vi "Corners to Rectangle.vi"(10 "Corners 2":cluster{"X":sgl, "Y":sgl}[](array[cluster])=[{"X"=418.12665, "Y"=424.52673}, {"X"=459.83737, "Y"=432.6989}, {"X"=455.7626, "Y"=481.78384}, {"X"=413.9875, "Y"=474.98163}, {"X"=418.12665, "Y"=424.52673}]) -> (2 "output cluster":T1, 4 "Aspect Ratio":sgl, 5 "Center":cluster{"X":dbl, "Y":dbl} {"Y" format="%0.2f"; "X" format="%0.2f"})   [LabVIEW 2023]
uses:
  Target Fields.ctl
  <vilib>/Analysis/baseanly.llb/Mean (DBL).vi
  <vilib>/Analysis/NI_AALBase.lvlib
panel:
  out "Tilted Left/Right":bool
  out "Tilted Up/down":bool
  out "Vert Size":sgl
  out "Horz Size":sgl
  out "Rectangle":T2
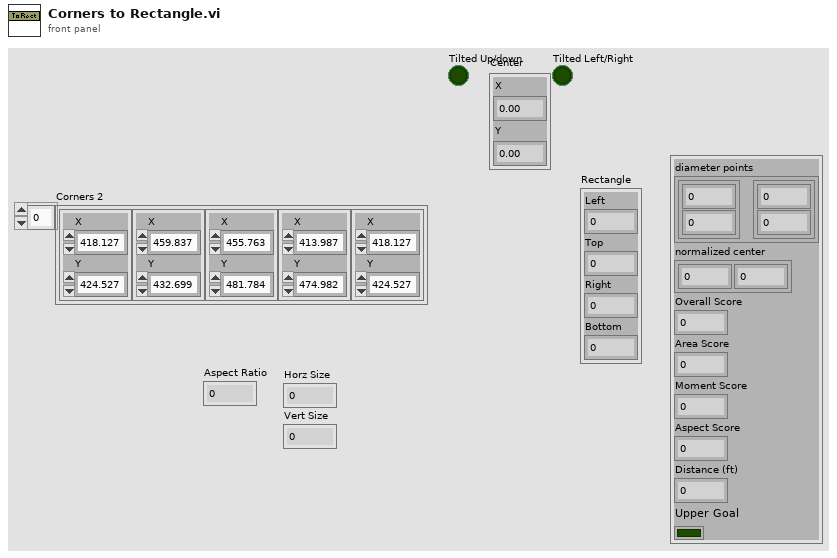
[diagram p1: front panel]
types:
  T1 = typedef "Target Fields.ctl" = cluster{"diameter points":cluster{"first point":cluster{"x":dbl, "y":dbl}, "projected point":cluster{"x":dbl, "y":dbl}}, "normalized center":cluster{"x":dbl, "y":dbl}, "Overall Score":dbl, "Area Score":dbl, "Moment Score":dbl, "Aspect Score":dbl, "Distance (ft)":dbl, "Upper Goal":bool}
  T2 = cluster{"Left":i32, "Top":i32, "Right":i32, "Bottom":i32}
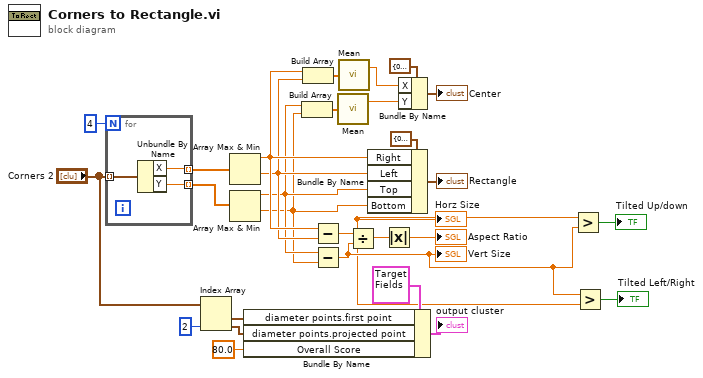
[diagram p0: block diagram]
diagram:
  n1 = for {
    N: 4 -> [_]
    tunnel: "Corners 2" -> [w31] mode=indexing
    tunnel: [w30] -> w28 mode=indexing
    tunnel: [w29] -> w27 mode=indexing
    n2 = Unbundle By Name(w31) -> ("X"=w30:sgl, "Y"=w29:sgl)
  }
  n3 = Index Array(array="Corners 2", index #2=2 ("index")) -> (element #1=w9:cluster{"X":sgl, "Y":sgl}, element #2=w8:cluster{"X":sgl, "Y":sgl})  [unwired: 1 in]
  n4 = Array Max & Min(array=w28) -> (max value=w21:sgl, min value=w20:sgl)  [unwired: 2 out]
  n5 = Array Max & Min(array=w27) -> (max value=w17:sgl, min value=w16:sgl)  [unwired: 2 out]
  n6 = Bundle By Name(cluster=T1 {"diameter points"={"first point"={"x"=0.0, "y"=0.0}, "projected point"={"x"=0.0, "y"=0.0}}, "normalized center"={"x"=0.0, "y"=0.0}, "Overall Score"=0.0, "Area Score"=0.0, "Moment Score"=0.0, "Aspect Score"=0.0, "Distance (ft)"=0.0, "Upper Goal"=FALSE} ("results"), "diameter points.first point"=w9, "diameter points.projected point"=w8, "Overall Score"=80.0) -> (→"output cluster":T1)
  n7 = Build Array(w17, w16) -> (w18:sgl[])
  n8 = Build Array(w21, w20) -> (w19:sgl[])
  n9 = Subtract(x=w21, y=w20) -> (x-y=w1:sgl)
  "Horz Size" <- w1
  n10 = Subtract(x=w17, y=w16) -> (x-y=w2:sgl)
  "Vert Size" <- w2
  n11 = call-poly <vilib>:"Mean.vi"("X"=w18) -> ("mean"=w13:dbl)  [unwired: 1 out]
  n12 = call-poly <vilib>:"Mean.vi"("X"=w19) -> ("mean"=w14:dbl)  [unwired: 1 out]
  n13 = Divide(x=w1, y=w2) -> (x/y=w23:sgl)
  n14 = Bundle By Name(cluster=T2 {"Left"=0, "Top"=0, "Right"=0, "Bottom"=0} ("Rectangle"), "Right"=w21, "Left"=w20, "Top"=w17, "Bottom"=w16) -> (→"Rectangle":T2)
  n15 = Absolute Value(x=w23) -> (abs(x)=→"Aspect Ratio":sgl)
  n16 = Bundle By Name(cluster=cluster{"X":dbl, "Y":dbl} {"X"=0.0, "Y"=0.0} ("Center"), "X"=w14, "Y"=w13) -> (→"Center":cluster{"X":dbl, "Y":dbl})
  n17 = Greater?(x=w1, y=w2) -> (0:→"Tilted Up/down":bool)
  n18 = Greater?(x=w2, y=w1) -> (0:→"Tilted Left/Right":bool)
